vi "example_usb.vi"() -> ()   [LabVIEW 2025, in "libirimager_direct_binding.lvlib"]
uses:
  libirimager_direct_binding.lvlib
panel:
  in  "transformation":T1(ring)
  out "Temp Graph":u32[][](graph)
  in  "palette (0...12)":i32
  in  "STOP Feed":bool
  in  "Focus Pos %":sgl min=0 max=100
  in  "setFocusPos":bool
  out "function return setFocusPos":i32
  out "function return set radiation":i32
  in  "tAmbient":sgl=-999.9 format="%#_6f"
  in  "transmissivity(0..1)":sgl=1.0 format="%#_6f"
  in  "emissivity(0..1)":sgl=1.0 format="%#_6f"
  in  "setRadiation":bool
  in  "STOP":bool
  out "Thermal Image":picture
  out "function return thm":i32
  out "thermal data out":u16[](array[numeric])
  out "function return savepng":i32
  in  "triggerFlag":bool
  out "function return triggerAutoflag":i32
  in  "set_trigger_mode":bool
  in  "state":i32
  out "function return setAutoflag":i32
  in  "terminate":bool
  out "function return terminate":i32
  in  "getThm":bool
  in  "connect_usb":bool
  in  "xml_camera_config":string="generic.xml"
  out "function return":i32
  out "w out":i32
  out "h out":i32
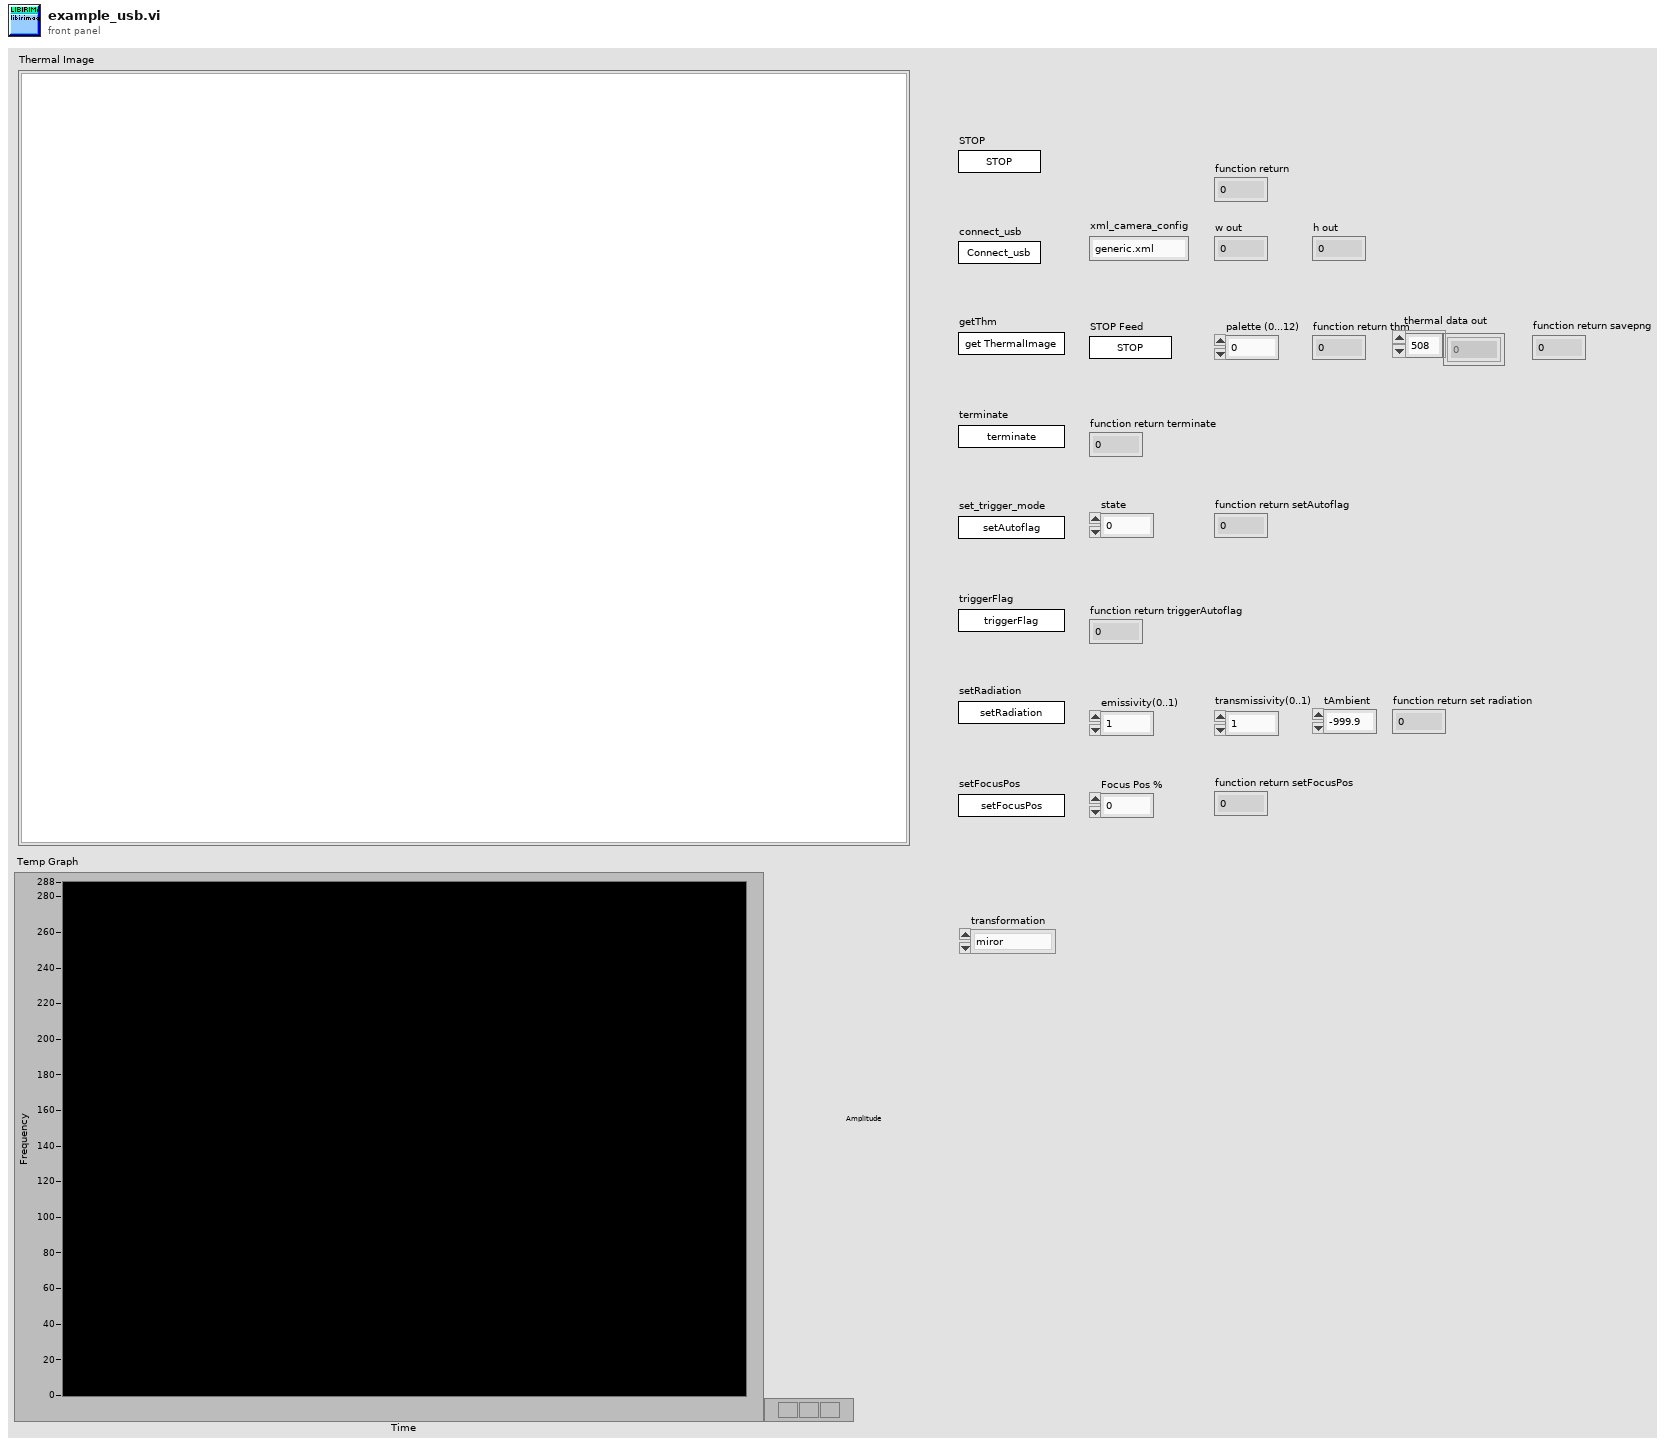
[diagram p1: front panel]
types:
  T1 = enum16{"miror", "rotate 0°", "rotate 90°", "rotate 180°", "rotate 270°"}
  T2 = typedef "LVBoundsTypeDef.ctl" = cluster{"Width":u32, "Height":u32}
  T3 = typedef "imagedata.ctl" = cluster{"image type":i32, "image depth":i32, "image":u8[], "mask":u8[], "colors":u32[], "Rectangle":cluster{"left":i16, "top":i16, "right":i16, "bottom":i16}}
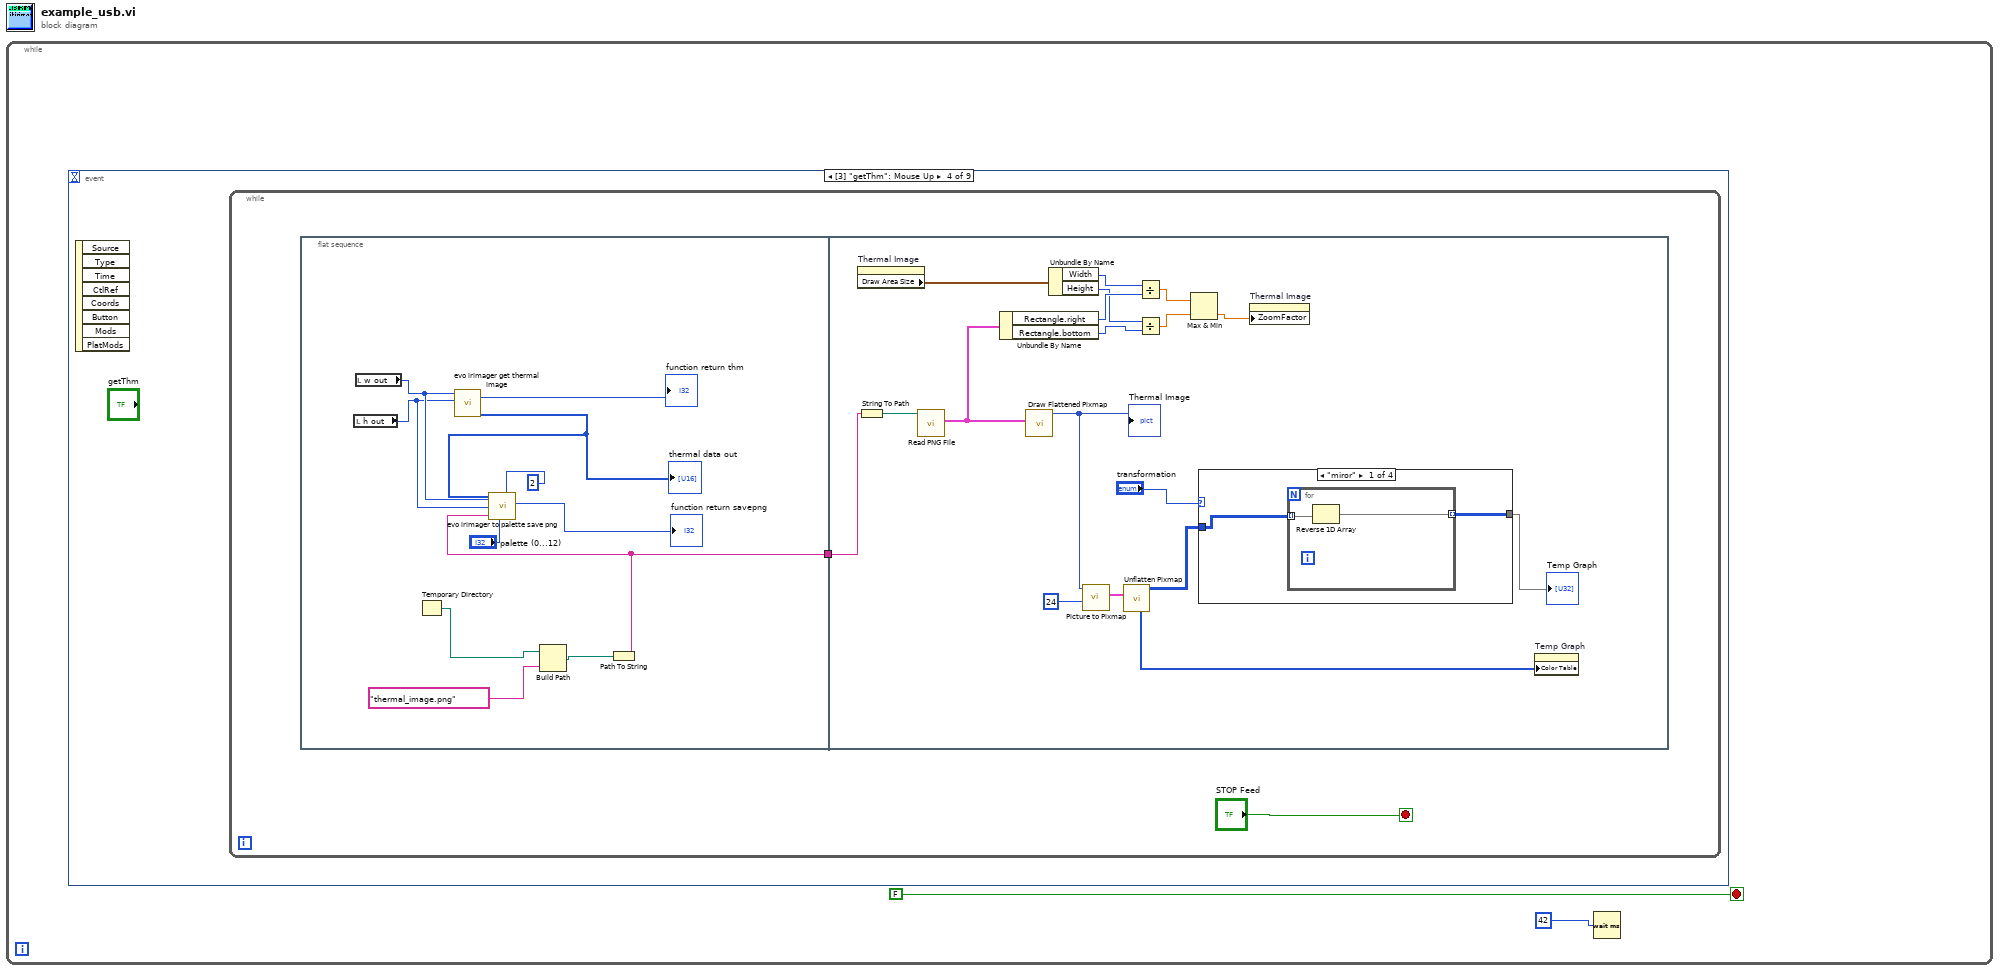
[diagram p0: block diagram]
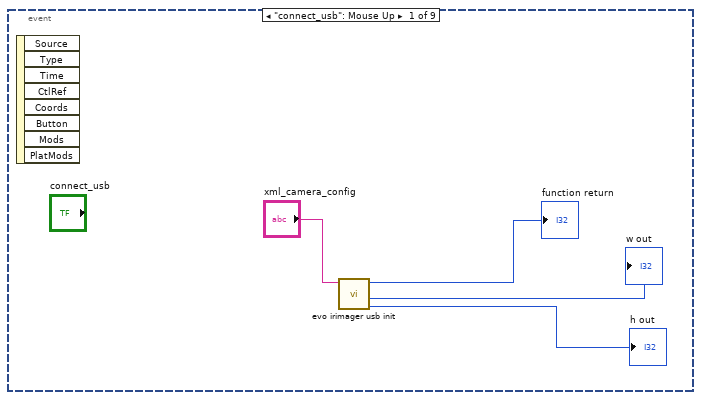
[diagram p2: hidden frame]
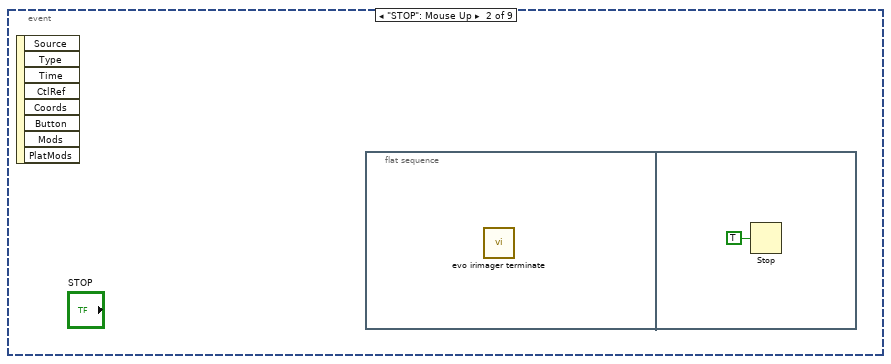
[diagram p3: hidden frame]
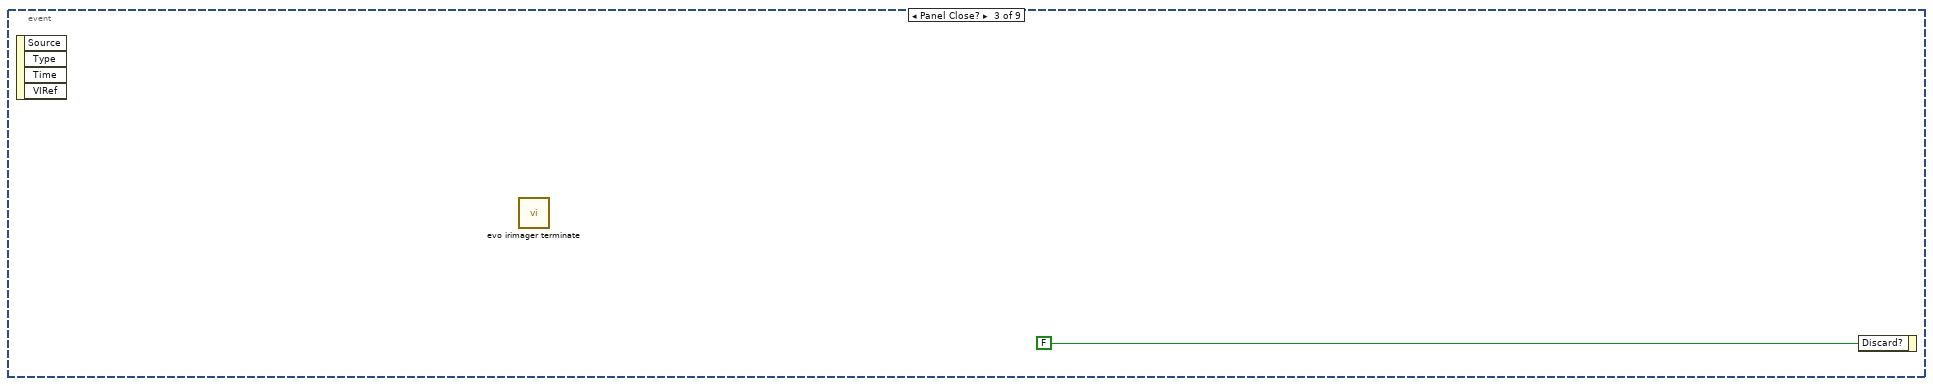
[diagram p4: hidden frame]
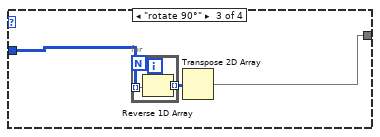
[diagram p6: hidden frame]
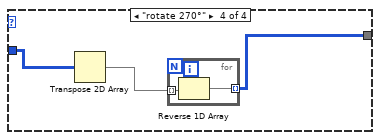
[diagram p7: hidden frame]
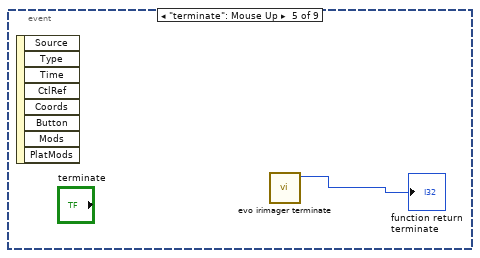
[diagram p8: hidden frame]
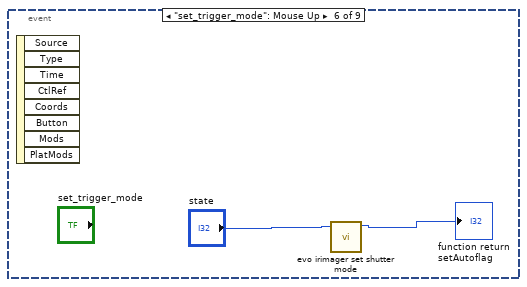
[diagram p9: hidden frame]
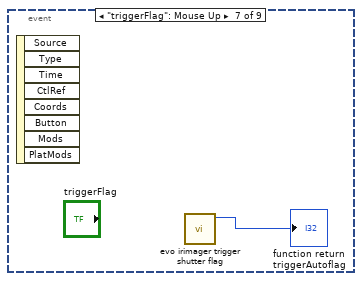
[diagram p10: hidden frame]
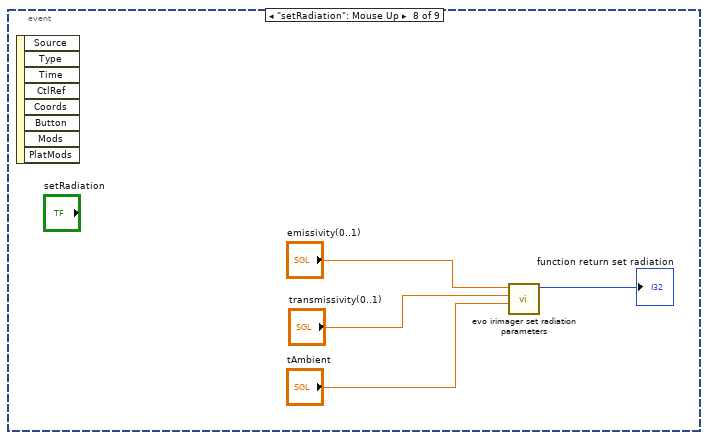
[diagram p11: hidden frame]
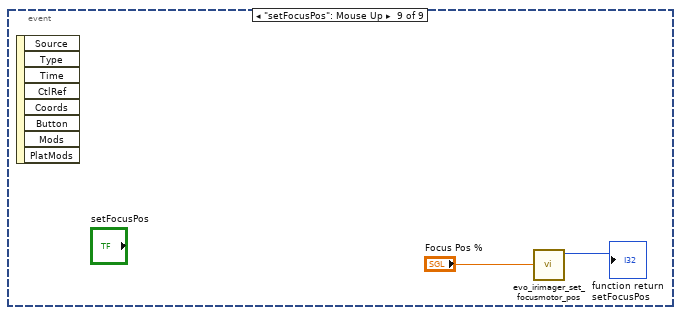
[diagram p12: hidden frame]
diagram:
  n1 = while {
    stop <- FALSE stop-if-true
    n2 = event shown="[3] \"getThm\": Mouse Up" {
      selector: _ -> [_ _ _ _ _ _ _ _ _]
      dyn-events: _ -> [_ _ _ _ _ _ _ _ _]
      timeout: _ -> [_ _ _ _ _ _ _ _ _]
      event "connect_usb": Mouse Up {
        n3 = event-data() -> ()  [unwired: 1 in, 8 out]
        n4 = call "evo irimager usb init.vi"("xml_config"="xml_camera_config") -> ("h out"=→"h out":i32, "w out"=→"w out":i32, "function return 2"=→"function return":i32)  [unwired: 7 in, 1 out]
      }
      event "STOP": Mouse Up {
        n5 = event-data() -> ()  [unwired: 1 in, 8 out]
        n6 = flat-sequence {
          frame #0 {
            n7 = call "evo irimager terminate.vi"() -> ()  [unwired: 11 in, 1 out]
          }
          frame #1 {
            n8 = Stop(stop? (T)=TRUE ("Stopp? (T)")) -> ()
          }
        }
      }
      event Panel Close? {
        n9 = event-data() -> ()  [unwired: 1 in, 4 out]
        n10 = call "evo irimager terminate.vi"() -> ()  [unwired: 11 in, 1 out]
        n11 = event-data("Discard?"=FALSE ("Verwerfen?")) -> ()  [unwired: 1 in, 1 out]
      }
      event "getThm": Mouse Up {
        n12 = event-data() -> ()  [unwired: 1 in, 8 out]
        n13 = while {
          stop <- "STOP Feed" stop-if-true
          n14 = flat-sequence {
            tunnel: [w14] -> w10
            tunnel: w10 -> [w38]
            frame #0 {
              n15 = local read "h out"() -> (w18:i32)
              n16 = local read "w out"() -> (w19:i32)
              n17 = Temporary Directory() -> (w13:path)
              n18 = call "evo irimager get thermal image.vi"("h"=w18, "w"=w19) -> ("data out"=w20:u16[], "function return"=→"function return thm":i32)  [unwired: 6 in, 2 out]
              "thermal data out" <- w20
              n19 = Build Path(base path=w13, name or relative path="thermal_image.png" ("String")) -> (appended path=w12:path)
              n20 = Path To String(path=w12) -> (string=w14:string)
              n21 = call "evo irimager to palette save png.vi"("palette_scale"=2, "palette"="palette (0...12)", "path"=w14, "h"=w18, "w"=w19, "thermal_data"=w20) -> ("function return"=→"function return savepng":i32)  [unwired: 4 in, 1 out]
            }
            frame #1 {
              n22 = property on="Thermal Image" class="Pict"() -> ("Draw Area Size"=w37:T2)  [unwired: 2 in, 2 out]
              n23 = String To Path(string=w38) -> (path=w39:path)
              n24 = call <vilib>:"Read PNG File.vi"("path to PNG file"=w39) -> ("image data"=w29:T3)  [unwired: 8 in, 2 out]
              n25 = Unbundle By Name(w29) -> ("Rectangle.right"=w36:i16, "Rectangle.bottom"=w33:i16)
              n26 = call <vilib>:"Draw Flattened Pixmap.vi"("image data"=w29) -> ("new picture"=w27:picture)  [unwired: 8 in]
              "Thermal Image" <- w27
              n27 = Unbundle By Name(w37) -> ("Width"=w35:u32, "Height"=w34:u32)
              n28 = call <vilib>:"Picture to Pixmap.vi"("depth"=24, "picture"=w27) -> ("image data"=w26:T3)  [unwired: 8 in, 1 out]
              n29 = call <vilib>:"Unflatten Pixmap.vi"("image data"=w26) -> ("24-bit pixmap"=w24:u32[][], "colors"=w22:u32[])  [unwired: 4 in, 5 out]
              n30 = Divide(x=w35, y=w36) -> (x/y=w32:dbl)
              n31 = Divide(x=w34, y=w33) -> (x/y=w31:dbl)
              n32 = Max & Min(x=w32, y=w31) -> (min(x,y)=w30:dbl)  [unwired: 1 out]
              n33 = case shown="\"miror\"" "transformation" {
                tunnel: w24 -> [w41 w44 w46 w51]
                tunnel: [w40 w44 w45 w50] -> w23
                frame "miror" {
                  n34 = for {
                    tunnel: w41 -> [w43] mode=indexing
                    tunnel: [w42] -> w40 mode=indexing
                    n35 = Reverse 1D Array(array=w43) -> (reversed array=w42:u32[])
                  }
                }
                frame "rotate 0°", Default {
                }
                frame "rotate 90°" {
                  n36 = for {
                    tunnel: w46 -> [w49] mode=indexing
                    tunnel: [w48] -> w47 mode=indexing
                    n37 = Reverse 1D Array(array=w49) -> (reversed array=w48:u32[])
                  }
                  n38 = Transpose 2D Array(2D array=w47) -> (transposed array=w45:u32[][])
                }
                frame "rotate 270°" {
                  n39 = Transpose 2D Array(2D array=w51) -> (transposed array=w52:u32[][])
                  n40 = for {
                    tunnel: w52 -> [w54] mode=indexing
                    tunnel: [w53] -> w50 mode=indexing
                    n41 = Reverse 1D Array(array=w54) -> (reversed array=w53:u32[])
                  }
                }
              }
              "Temp Graph" <- w23
              n42 = property on="Thermal Image" class="Pict"("ZoomFactor"=w30) -> ()  [unwired: 2 in, 2 out]
              n43 = property on="Temp Graph" class="IntChart (strict)"("Color Table"=w22) -> ()  [unwired: 2 in, 2 out]
            }
          }
        }
      }
      event "terminate": Mouse Up {
        n44 = event-data() -> ()  [unwired: 1 in, 8 out]
        n45 = call "evo irimager terminate.vi"() -> ("function return"=→"function return terminate":i32)  [unwired: 11 in]
      }
      event "set_trigger_mode": Mouse Up {
        n46 = event-data() -> ()  [unwired: 1 in, 8 out]
        n47 = call "evo irimager set shutter mode.vi"("mode"="state") -> ("function return"=→"function return setAutoflag":i32)  [unwired: 10 in]
      }
      event "triggerFlag": Mouse Up {
        n48 = event-data() -> ()  [unwired: 1 in, 8 out]
        n49 = call "evo irimager trigger shutter flag.vi"() -> ("function return"=→"function return triggerAutoflag":i32)  [unwired: 11 in]
      }
      event "setRadiation": Mouse Up {
        n50 = event-data() -> ()  [unwired: 1 in, 8 out]
        n51 = call "evo irimager set radiation parameters.vi"("tAmbient"="tAmbient", "transmissivity"="transmissivity(0..1)", "emissivity"="emissivity(0..1)") -> ("function return"=→"function return set radiation":i32)  [unwired: 8 in]
      }
      event "setFocusPos": Mouse Up {
        n52 = event-data() -> ()  [unwired: 1 in, 8 out]
        n53 = call "evo_irimager_set_focusmotor_pos.vi"("Focus Pos %"="Focus Pos %") -> ("function return"=→"function return setFocusPos":i32)  [unwired: 10 in]
      }
    }
    n54 = Wait (ms)(milliseconds to wait=u32 42) -> ()  [unwired: 1 out]
  }
